vi "login2.vi"() -> ()   [LabVIEW 2017]
panel:
  in  "Password":string
  in  "Login":string
  out "Boolean 2":bool
  out "Boolean":bool
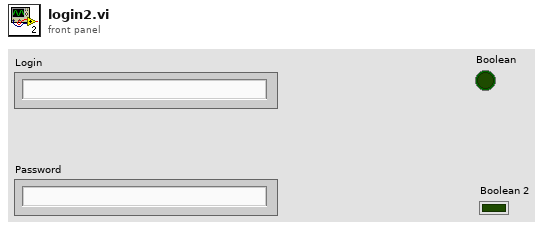
[diagram p1: front panel]
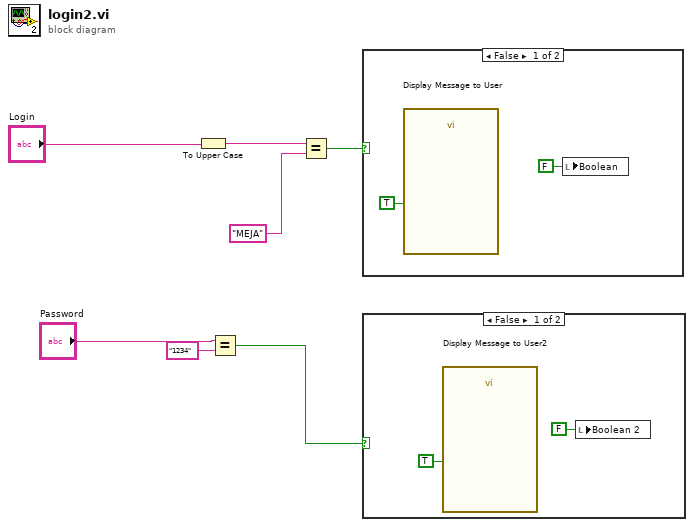
[diagram p0: block diagram]
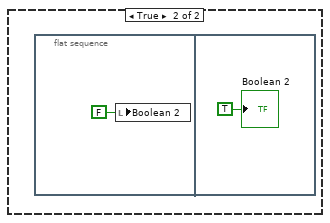
[diagram p2: hidden frame]
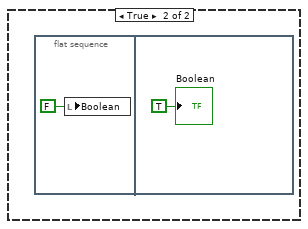
[diagram p3: hidden frame]
diagram:
  n1 = To Upper Case(1:"Login") -> (0:w4:string)
  n2 = Equal?(x="Password", y="1234") -> (x = y?=w6:bool)
  n3 = Equal?(x=w4, y="MEJA") -> (x = y?=w7:bool)
  n4 = case shown="False" w7 {
    frame False {
      n5 = call "Display Message to User"("Enable"=TRUE) -> ()  [unwired: 9 in, 2 out]
      n6 = local write "Boolean"(FALSE ("Boolean")) -> ()
    }
    frame True {
      n7 = flat-sequence {
        frame #0 {
          n8 = local write "Boolean"(FALSE ("Boolean")) -> ()
        }
        frame #1 {
          "Boolean" <- TRUE ("Boolean")
        }
      }
    }
  }
  n9 = case shown="False" w6 {
    frame False {
      n10 = call "Display Message to User2"("Enable"=TRUE) -> ()  [unwired: 9 in, 2 out]
      n11 = local write "Boolean 2"(FALSE ("Boolean 2")) -> ()
    }
    frame True {
      n12 = flat-sequence {
        frame #0 {
          n13 = local write "Boolean 2"(FALSE ("Boolean 2")) -> ()
        }
        frame #1 {
          "Boolean 2" <- TRUE ("Boolean 2")
        }
      }
    }
  }
